vi "Test WS5100.vi"() -> ()   [LabVIEW 2020, in "WS5100.lvclass"]
uses:
  WS5100.lvclass
  Controls/Change setting mode enum.ctl
  PIC-device/PIC-Device.lvclass
panel:
  out "Changes":cluster{"Name":string, "Value":string}[][](array[cluster])
  in  "y":bool
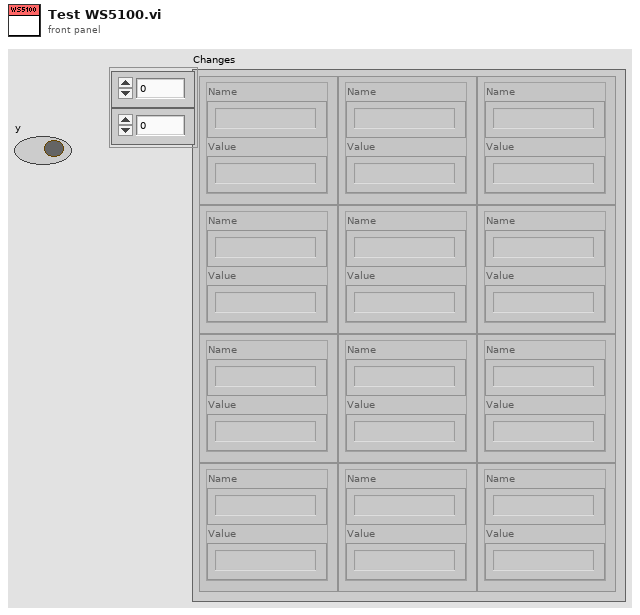
[diagram p1: front panel]
types:
  T1 = typedef "PIC-Device.lvclass/Change setting mode enum.ctl" = enum16{"Init", "Next", "Reset"}
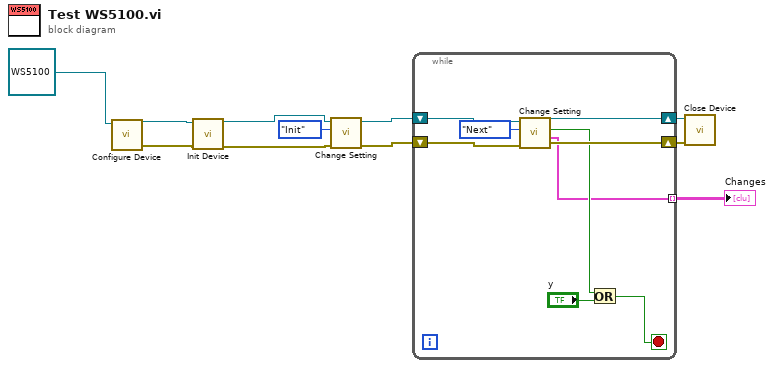
[diagram p0: block diagram]
diagram:
  n1 = call-dynamic "Configure Device.vi"("WS5100 in"=refnum<class "WS5100.lvclass"> refnum ("WS5100.lvclass")) -> ("error out"=w4:errorcluster, "WS5100 out"=w3:refnum<class "WS5100.lvclass">)  [unwired: 9 in]
  n2 = call-dynamic "Init Device.vi"("error in (no error)"=w4, "NI DAQmx in"=w3) -> ("error out"=w2:errorcluster, "NI DAQmx out"=w1:refnum<class "WS5100.lvclass">)  [unwired: 8 in]
  n3 = call-dynamic "Change Setting.vi"("error in (no error)"=w2, "Change setting mode"=Change_setting_mode_enum."Init", "NI DAQmx in"=w1) -> ("error out"=w9:errorcluster, "NI DAQmx out"=w10:refnum<class "WS5100.lvclass">)  [unwired: 5 in, 2 out]
  n4 = while {
    shift-right: [w18] -> w8
    shift-left: w10 -> [w20]
    shift-right: [w17] -> w7
    shift-left: w9 -> [w19]
    tunnel: [w12] -> w5 mode=indexing
    stop <- w13 stop-if-true
    n5 = call-dynamic "Change Setting.vi"("error in (no error)"=w19, "Change setting mode"=Change_setting_mode_enum."Next", "NI DAQmx in"=w20) -> ("error out"=w17:errorcluster, "Changes"=w12:cluster{"Name":string, "Value":string}[], "Last setting"=w15:bool, "NI DAQmx out"=w18:refnum<class "WS5100.lvclass">)  [unwired: 5 in]
    n6 = Or(x=w15, y="y") -> (x .or. y?=w13:bool)
  }
  "Changes" <- w5
  n7 = call-dynamic "Close Device.vi"("error in (no error)"=w7, "NI DAQmx in"=w8) -> ()  [unwired: 8 in, 2 out]
